vi "SHA-2-U64.vi"(7 "Type":T1, 8 "error in (no error)":errorcluster, 11 "Message":u8[](array[numeric])) -> (0 "error out":errorcluster, 1 "ASCII Formatted hash":string, 3 "binary string hash":u8[](array[numeric]) caption="Hash")   [LabVIEW 2011, in "i3-external-encryption.lvlib"]
doc: "Performs an SHA2 U64-bit.\n\n(c) Ton Plomp, 2011\nTHIS SOFTWARE IS PROVIDED AS IS, AND ANY WARRANTY IS REJECTED"
uses:
  i3-external-encryption.lvlib
  SHA-2_U64_types.ctl
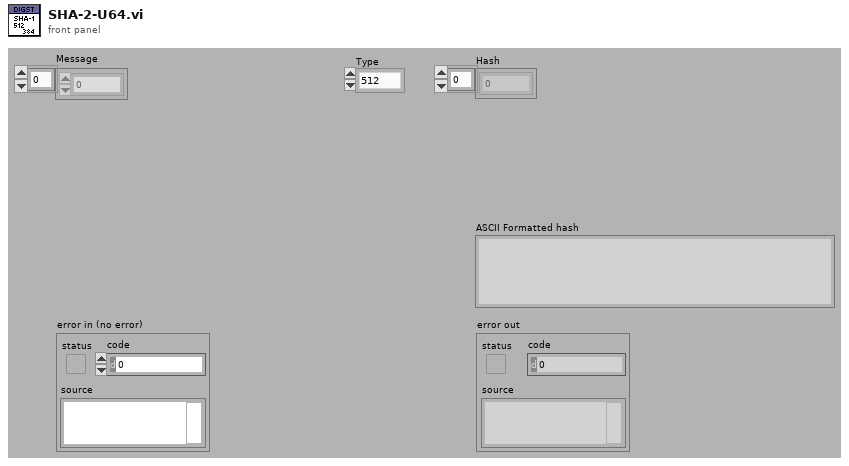
[diagram p1: front panel]
types:
  T1 = typedef "i3-external-encryption.lvlib/SHA-2_U64_types.ctl" = enum16{"512", "384"}
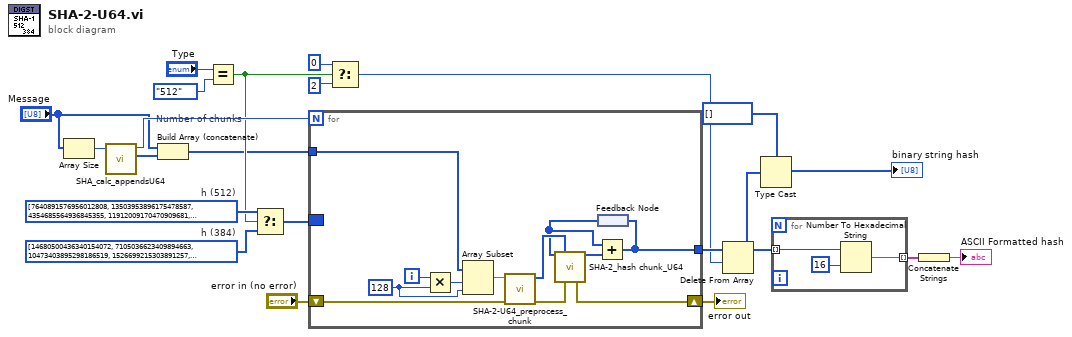
[diagram p0: block diagram]
diagram:
  w11 = u64[] [14680500436340154072, 7105036623409894663, 10473403895298186519, 1526699215303891257, 7436329637833083697, 10282925794625328401, 15784041429090275239, 5167115440072839076]  # h (384)
  w15 = u64[] [7640891576956012808, 13503953896175478587, 4354685564936845355, 11912009170470909681, 5840696475078001361, 11170449401992604703, 2270897969802886507, 6620516959819538809]  # h (512)
  # "Number of chunks"
  n1 = Array Size(array="Message") -> (size(s)=w7:i32)
  n2 = call "SHA_calc_appendsU64.vi"("String length"=w7) -> ("Append"=w6:u8[], "Number of chunks"=w22:i32)  [unwired: 9 in]
  n3 = Build Array (concatenate)("Message", w6) -> (w4:u8[])
  n4 = Equal?(x="Type", y=SHA-2_U64_types."512" ("Type")) -> (x = y?=w12:bool)
  n5 = Select(t=w15, s=w12, f=w11) -> (s? t:f=w14:u64[])
  n6 = for {
    N: w22 -> [_]
    tunnel: w4 -> [w34]
    tunnel: [w25] -> w13
    border: w14 -> [_]
    shift-right: [w29] -> w21
    shift-left: "error in (no error)" -> [w28]
    i -> [w31]
    w32 = 128 ("x")
    n7 = Multiply(x=w31, y=w32) -> (x*y=w33:i32)
    n8 = Array Subset(array=w34, index=w33, length=w32) -> (w23:u8[])
    n9 = call "SHA-2-U64_preprocess_chunk.vi"("error in (no error)"=w28, "Chunk in"=w23) -> ("error out"=w26:errorcluster, "Processed chunk out"=w27:u64[])  [unwired: 8 in]
    n10 = feedback #1() -> (w24:u64[])
    n11 = call "SHA-2_hash chunk_U64.vi"("h in"=w24, "Chunk"=w27, "error in (no error)"=w26) -> ("h out"=w30:u64[], "error out"=w29:errorcluster)  [unwired: 11 in]
    n12 = Add(x=w24, y=w30) -> (x+y=w25:u64[])
    n13 = feedback-in #1(w25) -> ()
  }
  "error out" <- w21
  n14 = Select(t=0, s=w12, f=2 ("length")) -> (s? t:f=w8:i32)
  n15 = Delete From Array(array=w13, length=w8) -> (array with subset deleted=w1:u64[])  [unwired: 1 in, 1 out]
  n16 = Type Cast(type=u8[] [] ("binary string hash"), x=w1) -> (*(type *) &x=→"binary string hash":u8[])
  n17 = for {
    tunnel: w1 -> [w37] mode=indexing
    tunnel: [w35] -> w19 mode=indexing
    n18 = Number To Hexadecimal String(1:i16 16 ("width (-)"), 2:w37) -> (0:w35:string)
  }
  n19 = Concatenate Strings(w19) -> (→"ASCII Formatted hash":string)
